vi "Machine Cal Data Engine.vi"   [LabVIEW 2019]
uses:
  Type Defs/TCP Data Stream Mode (PC).ctl
types:
  T1 = typedef "TCP Data Stream Mode (PC).ctl" = enum16{"Init", "Read Data", "Close"}
  T2 = enum16{"Init", "Start Data", "Stop Data", "Lost Connection", "Engine Idle", "Write Data", "Read Data"}
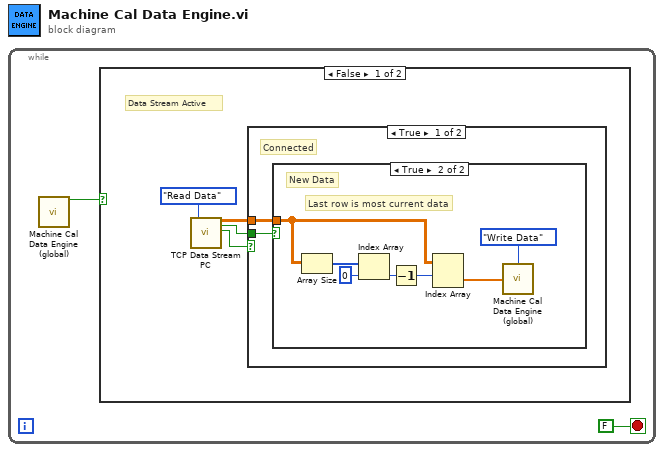
[diagram p0: block diagram]
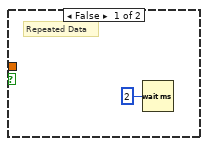
[diagram p2: hidden frame]
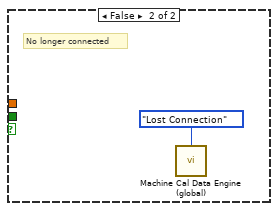
[diagram p3: hidden frame]
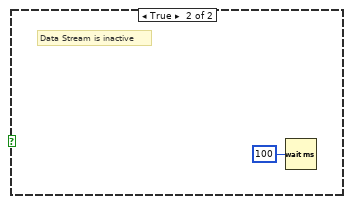
[diagram p4: hidden frame]
diagram:
  n1 = while {
    stop <- FALSE stop-if-true
    n2 = call "Machine Cal Data Engine (global).vi"() -> ("Stream Data"=w1:bool)  [unwired: 12 in, 3 out]
    n3 = case shown="False" w1 {
      frame False {
        # "Data Stream Active"
        n4 = call "TCP Data Stream PC.vi"("Mode"=TCP_Data_Stream_Mode_(PC)."Read Data") -> ("Data OUT"=w3:dbl[][], "New Data?"=w4:bool, "Connected?"=w5:bool)  [unwired: 15 in, 1 out]
        n5 = case shown="True" w5 {
          tunnel: w4 -> [w8 _]
          tunnel: w3 -> [w7 _]
          frame True {
            # "Connected"
            n6 = case shown="True" w8 {
              tunnel: w7 -> [_ w15]
              frame False {
                # "Repeated Data"
                n7 = Wait (ms)(milliseconds to wait=u32 2) -> ()  [unwired: 1 out]
              }
              frame True {
                # "Last row is most current data"
                # "New Data"
                n8 = Array Size(array=w15) -> (size(s)=w14:i32[])
                n9 = Index Array(array=w14, index=0) -> (element=w12:i32)
                n10 = Decrement(x=w12) -> (x-1=w11:i32)
                n11 = Index Array(array=w15, index (row)=w11) -> (element=w10:dbl[])  [unwired: 1 in]
                n12 = call "Machine Cal Data Engine (global).vi"("Mode"=T2."Write Data", "Data In"=w10) -> ()  [unwired: 10 in, 4 out]
              }
            }
          }
          frame False {
            # "No longer connected"
            n13 = call "Machine Cal Data Engine (global).vi"("Mode"=T2."Lost Connection") -> ()  [unwired: 11 in, 4 out]
          }
        }
      }
      frame True {
        # "Data Stream is inactive"
        n14 = Wait (ms)(milliseconds to wait=u32 100) -> ()  [unwired: 1 out]
      }
    }
  }
